vi "SimpleDemo.vi"() -> ()   [LabVIEW 2011]
panel:
  out "NumPoints":i32
  out "XY Graph":cluster{dbl[], dbl[]}(graph)
  out "error out":errorcluster
  in  "SampleRate":sgl=0.1
  in  "Tfinal":sgl=1.0
  in  "Vfinal":sgl=-0.1
  in  "Tinit":sgl=1.0
  in  "Vinit":sgl=0.1
  in  "GAMRYCOMLib.IGamrySignal":refnum<k7>
  in  "GAMRYCOMLib.IGamrySignalStep":refnum<k7>
  in  "GAMRYCOMLib.IGamryDtaqIv":refnum<k7>
  in  "GAMRYCOMLib.IGamryPstat":refnum<k7>
  in  "GAMRYCOMLib.IGamryDeviceList":refnum<k7>
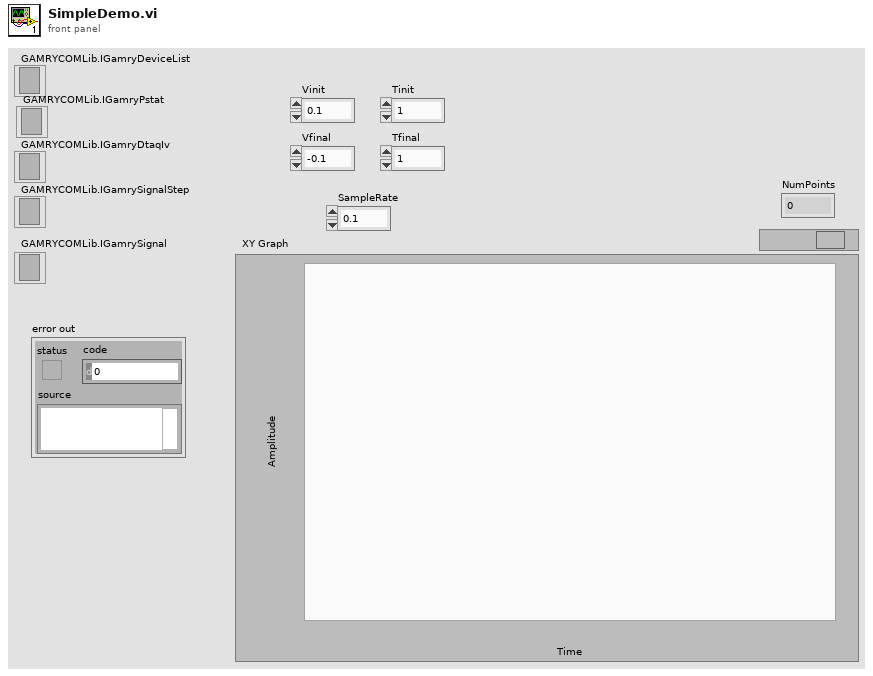
[diagram p1: front panel]
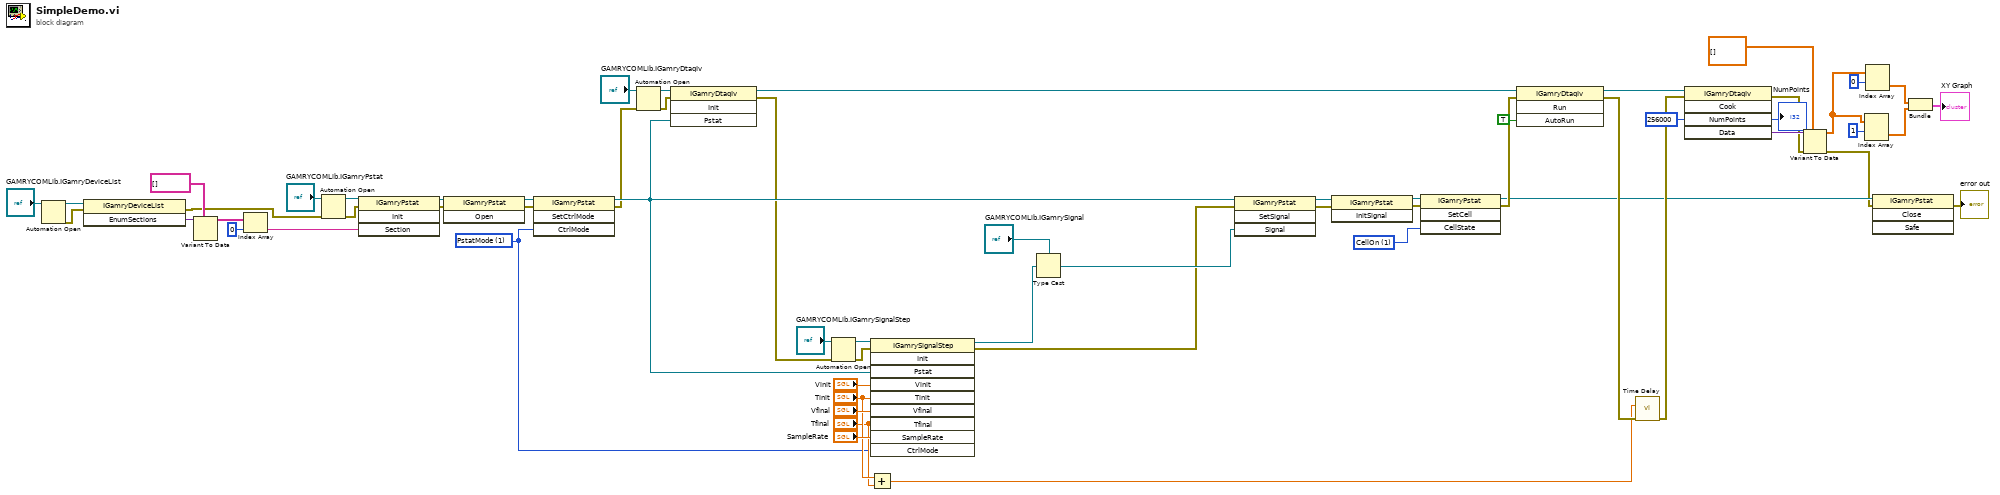
[diagram p0: block diagram]
diagram:
  w31 = 1 items=["CellOff", "CellOn", "CellMon", "CellRelay"] ("CellState")
  w2 = 1 items=["GstatMode", "PstatMode", "ZRAMode", "FRAMode"] ("CtrlMode")
  n1 = Automation Open(Automation Refnum="GAMRYCOMLib.IGamryDeviceList") -> (Automation Refnum=w60:refnum<k7>, error out=w59:errorcluster)  [unwired: 3 in]
  n2 = invoke class="IGamryDeviceList" method="EnumSections"(reference=w60, error in=w59) -> (error out=w45:errorcluster, "EnumSections"=w58:variant)  [unwired: 1 in, 1 out]
  n3 = Variant To Data(type=string[] [], Variant=w58) -> (data=w56:string[])  [unwired: 1 in, 1 out]
  n4 = Index Array(array=w56, index=0) -> (element=w51:string)
  n5 = Automation Open(error in (no error)=w45, Automation Refnum="GAMRYCOMLib.IGamryPstat") -> (Automation Refnum=w53:refnum<k7>, error out=w52:errorcluster)  [unwired: 2 in]
  n6 = invoke class="IGamryPstat" method="Init"(reference=w53, error in=w52, "Section"=w51) -> (reference out=w49:refnum<k7>, error out=w50:errorcluster)  [unwired: 1 in, 2 out]
  n7 = invoke class="IGamryPstat" method="Open"(reference=w49, error in=w50) -> (reference out=w41:refnum<k7>, error out=w40:errorcluster)  [unwired: 1 in, 1 out]
  n8 = invoke class="IGamryPstat" method="SetCtrlMode"(reference=w41, error in=w40, "CtrlMode"=w2) -> (reference out=w39:refnum<k7>, error out=w28:errorcluster)  [unwired: 1 in, 2 out]
  n9 = Automation Open(error in (no error)=w28, Automation Refnum="GAMRYCOMLib.IGamryDtaqIv") -> (Automation Refnum=w47:refnum<k7>, error out=w46:errorcluster)  [unwired: 2 in]
  n10 = invoke class="IGamryDtaqIv" method="Init"(reference=w47, error in=w46, "Pstat"=w39) -> (reference out=w30:refnum<k7>, error out=w27:errorcluster)  [unwired: 1 in, 2 out]
  n11 = Automation Open(error in (no error)=w27, Automation Refnum="GAMRYCOMLib.IGamrySignalStep") -> (Automation Refnum=w43:refnum<k7>, error out=w42:errorcluster)  [unwired: 2 in]
  n12 = Add(x="Tinit", y="Tfinal") -> (x+y=w19:sgl)
  n13 = invoke class="IGamrySignalStep" method="Init"(reference=w43, error in=w42, "Pstat"=w39, "Vinit"="Vinit", "Tinit"="Tinit", "Vfinal"="Vfinal", "Tfinal"="Tfinal", "SampleRate"="SampleRate", "CtrlMode"=w2) -> (reference out=w38:refnum<k7>, error out=w26:errorcluster)  [unwired: 1 in, 8 out]
  n14 = Type Cast(type="GAMRYCOMLib.IGamrySignal", x=w38) -> (*(type *) &x=w36:refnum<k7>)
  n15 = invoke class="IGamryPstat" method="SetSignal"(reference=w39, error in=w26, "Signal"=w36) -> (reference out=w35:refnum<k7>, error out=w34:errorcluster)  [unwired: 1 in, 2 out]
  n16 = invoke class="IGamryPstat" method="InitSignal"(reference=w35, error in=w34) -> (reference out=w33:refnum<k7>, error out=w32:errorcluster)  [unwired: 1 in, 1 out]
  n17 = invoke class="IGamryPstat" method="SetCell"(reference=w33, error in=w32, "CellState"=w31) -> (reference out=w15:refnum<k7>, error out=w29:errorcluster)  [unwired: 1 in, 2 out]
  n18 = invoke class="IGamryDtaqIv" method="Run"(reference=w30, error in=w29, "AutoRun"=TRUE) -> (reference out=w17:refnum<k7>, error out=w22:errorcluster)  [unwired: 1 in, 2 out]
  n19 = call "Time Delay"("error in (no error)"=w22, "Delay Time (s)"=w19) -> ("error out"=w18:errorcluster)  [unwired: 9 in]
  n20 = invoke class="IGamryDtaqIv" method="Cook"(reference=w17, error in=w18, "NumPoints"=256000) -> (error out=w12:errorcluster, "NumPoints"=→"NumPoints":i32, "Data"=w13:variant)  [unwired: 2 in, 2 out]
  n21 = Variant To Data(error in=w12, type=dbl[][] [], Variant=w13) -> (data=w7:dbl[][], error out=w11:errorcluster)
  n22 = Index Array(array=w7, index (row)=1) -> (element=w5:dbl[])  [unwired: 1 in]
  n23 = Index Array(array=w7, index (row)=0) -> (element=w6:dbl[])  [unwired: 1 in]
  n24 = invoke class="IGamryPstat" method="Close"(reference=w15, error in=w11) -> (error out=→"error out":errorcluster)  [unwired: 2 in, 3 out]
  n25 = Bundle(w6, w5) -> (→"XY Graph":cluster{dbl[], dbl[]})  [unwired: 1 in]
